vi "Write Auto Load.vi"(8 "error in (no error)":errorcluster, 10 "Auto Load":bool, 11 "ProjectLoader in":refnum<class "ProjectLoader.lvclass">) -> (0 "error out":errorcluster, 3 "ProjectLoader out":refnum<class "ProjectLoader.lvclass">)   [LabVIEW 2015, in "ProjectLoader.lvclass"]
uses:
  ProjectLoader.lvclass
  ProjectLoader.lvclass/ProjectLoader.ctl
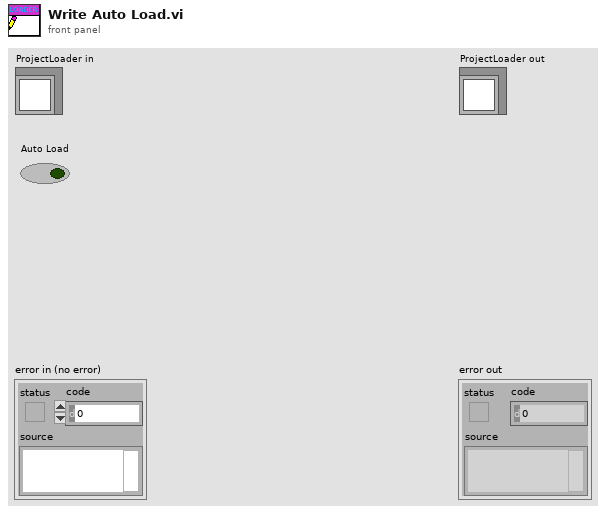
[diagram p1: front panel]
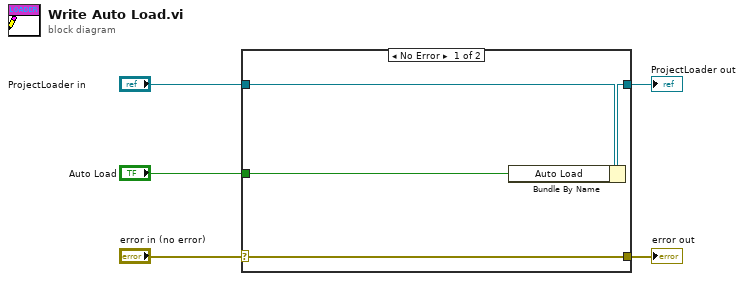
[diagram p0: block diagram]
diagram:
  n1 = case shown="No Error" "error in (no error)" {
    selector: "error in (no error)" -> [w9 w10]
    tunnel: [w9 w10] -> w4
    tunnel: [w7 w11] -> w2
    tunnel: "ProjectLoader in" -> [w8 w11]
    tunnel: "Auto Load" -> [w6 _]
    frame No Error {
      n2 = Bundle By Name(cluster=w8, "Auto Load"=w6) -> (w7:refnum<class "ProjectLoader.lvclass">)
    }
    frame Error {
    }
  }
  "error out" <- w4
  "ProjectLoader out" <- w2
